vi "inclinometer_model.vi"(10 "input_signal(V)":dbl) -> (2 "output_angle(deg)":dbl)   [LabVIEW 2020]
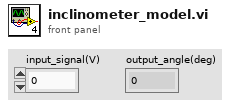
[diagram p1: front panel]
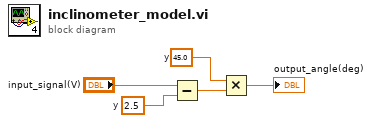
[diagram p0: block diagram]
diagram:
  w5 = 2.5  # y
  w4 = 45.0  # y
  n1 = Subtract(x="input_signal(V)", y=w5) -> (x-y=w2:dbl)
  n2 = Multiply(x=w4, y=w2) -> (x*y=→"output_angle(deg)":dbl)
